vi "GetHybridNodeTOF.vi"() -> (0 "TOF Valid [t0]":bool, 1 "Hybrid Node Range (in) [t0]":dbl)   [LabVIEW 2020]
doc: "Gets the current reading from the hybrid node time-of-flight sensor and performs validity checks."
uses:
  <vilib>/Playing With Fusion Inc/Playing With Fusion Lib for FRC/PWF_ToF_LabVIEW/Public/TypeDefs/PwF_ToF_Status.ctl
  <vilib>/Playing With Fusion Inc/Playing With Fusion Lib for FRC/PWF_ToF_LabVIEW/PwF_ToF.lvlib
  GlobalMiscellaneous.vi
  62455354-eac0-4b39-8d8a-3ef8c322dc59.vi
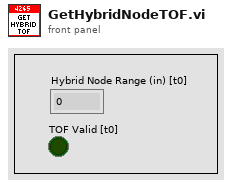
[diagram p1: front panel]
types:
  T1 = typedef "PlayingWithFusionLib.lvlib/PwF_ToF.lvlib/PwF_ToF_Status.ctl" = u16
  T2 = typedef "PlayingWithFusionLib.lvlib/PwF_ToF.lvlib/PwF_ToF_DevRef.ctl" = cluster{"DeviceStatus":errorcluster, "Device Number":u8, "Handle":u64, "Library Path":path}
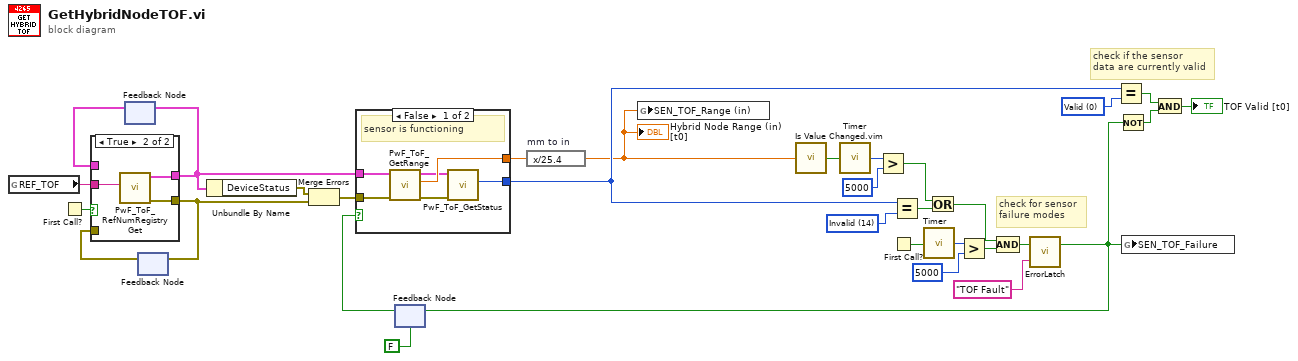
[diagram p0: block diagram]
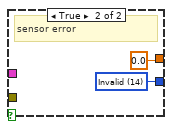
[diagram p3: hidden frame]
diagram:
  w20 = T1 0 items=["Valid"=0, "SigmaHigh"=1, "ReturnSignalLow"=2, "ReturnPhaseBad"=4, "HardwareFailure"=5, "WrappedTarget"=7, "InternalError"=8, "Invalid"=14] ("y")
  w22 = T1 14 items=["Valid"=0, "SigmaHigh"=1, "ReturnSignalLow"=2, "ReturnPhaseBad"=4, "HardwareFailure"=5, "WrappedTarget"=7, "InternalError"=8, "Invalid"=14] ("y")
  # "check if the sensor\ndata are currently valid"
  # "check for sensor\nfailure modes"
  n1 = global read "GlobalMiscellaneous.vi" "REF_TOF"() -> (w3:string)
  n2 = First Call?() -> (First Call?: T/F=w8:bool)
  n3 = feedback #1() -> (w7:T2)  [unwired: 1 in]
  n4 = feedback #2() -> (w6:errorcluster)  [unwired: 1 in]
  n5 = case shown="True" w8 {
    tunnel: [w33 w36] -> w1
    tunnel: w7 -> [w33 _]
    tunnel: [w32 w35] -> w4
    tunnel: w6 -> [w32 _]
    tunnel: w3 -> [_ w34]
    frame False {
    }
    frame True {
      n6 = call <vilib>:"PwF_ToF_RefNumRegistryGet.vi"("refnum name"=w34) -> ("error out"=w35:errorcluster, "PwFToFDevRefOut"=w36:T2)  [unwired: 9 in]
    }
  }
  n7 = feedback-in #1(w1) -> ()
  n8 = feedback-in #2(w4) -> ()
  n9 = Unbundle By Name(w1) -> ("DeviceStatus"=w5:errorcluster)
  n10 = Merge Errors(w5, w4) -> (w2:errorcluster)
  n11 = feedback #3(FALSE ("Latched")) -> (w24:bool)
  n12 = case shown="False" w24 {
    tunnel: [w42 0.0 ("range (mm)")] -> w14
    tunnel: [w39 w44] -> w21
    tunnel: w2 -> [w38 _]
    tunnel: w1 -> [w37 _]
    frame False {
      # "sensor is functioning"
      n13 = call <vilib>:"PwF_ToF_GetRange.vi"("error in"=w38, "PwFToFDevRefIn"=w37) -> ("error out"=w40:errorcluster, "range (mm)"=w42:dbl, "PwFToFDevRefOut"=w41:T2)  [unwired: 7 in]
      n14 = call <vilib>:"PwF_ToF_GetStatus.vi"("error in"=w40, "PwFToFDevRefIn"=w41) -> ("status"=w39:T1)  [unwired: 7 in, 2 out]
    }
    frame True {
      w44 = T1 14 items=["Valid"=0, "SigmaHigh"=1, "ReturnSignalLow"=2, "ReturnPhaseBad"=4, "HardwareFailure"=5, "WrappedTarget"=7, "InternalError"=8, "Invalid"=14] ("status")
      # "sensor error"
    }
  }
  n15 = expression code="x/25.4" "mm to in"(w14) -> (w13:dbl)
  "Hybrid Node Range (in) [t0]" <- w13
  n16 = global write "GlobalMiscellaneous.vi" "SEN_TOF_Range (in)"(w13) -> ()
  n17 = call "Is Value Changed.vim"("value"=w13) -> ("changed or first call?"=w19:bool)
  n18 = call "Timer.vi"("Reset Timer"=w19) -> ("Time (ms)"=w18:u32)
  n19 = Greater?(x=w18, y=u32 5000) -> (0:w15:bool)
  n20 = First Call?() -> (First Call?: T/F=w27:bool)
  n21 = Equal?(x=w21, y=w22) -> (x = y?=w25:bool)
  n22 = call "Timer.vi"("Reset Timer"=w27) -> ("Time (ms)"=w31:u32)
  n23 = Or(x=w15, y=w25) -> (x .or. y?=w16:bool)
  n24 = Greater?(x=w31, y=u32 5000) -> (0:w29:bool)
  n25 = Compound Arithmetic op=AND(w16, w29) -> (w26:bool)
  n26 = call "ErrorLatch.vi"("Error Message"="TOF Fault", "Trigger"=w26) -> ("Latched"=w10:bool)  [unwired: 1 in]
  n27 = feedback-in #3(w10) -> ()
  n28 = Equal?(x=w21, y=w20) -> (x = y?=w9:bool)
  n29 = Not(x=w10) -> (.not. x?=w11:bool)
  n30 = global write "GlobalMiscellaneous.vi" "SEN_TOF_Failure"(w10) -> ()
  n31 = And(x=w9, y=w11) -> (x .and. y?=→"TOF Valid [t0]":bool)
